vi "sortTimes.vi"(8 "error in (no error)":errorcluster, 10 "Array":T2(array[cluster]), 11 "ScriptEventList in":refnum<class "ScriptEventList.lvclass">) -> (0 "error out":errorcluster, 2 "sortedData":T1, 3 "ScriptEventList out":refnum<class "ScriptEventList.lvclass">)   [LabVIEW 2009, in "Tools.lvlib" / "Scripting.lvlib" / "ScriptEventList.lvclass"]
uses:
  ScriptEventList.lvclass
  DatabaseHelpers/Database Objects/Channel/Channel.lvclass
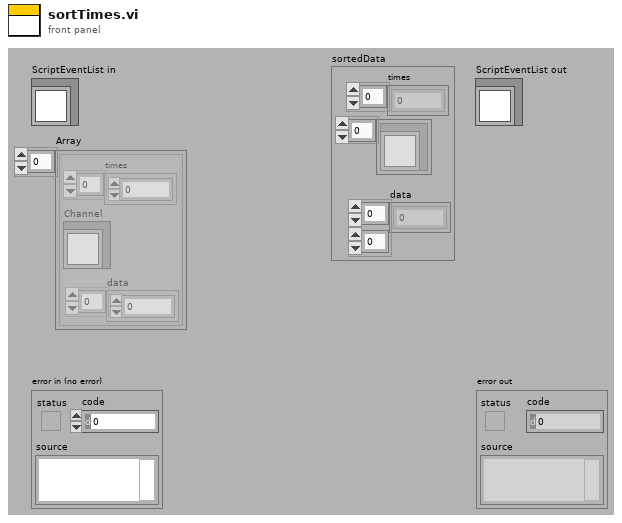
[diagram p1: front panel]
types:
  T1 = cluster{"times":dbl[], refnum<class "Channel.lvclass">[], "data":dbl[][]}
  T2 = cluster{"times":dbl[], "Channel":refnum<class "Channel.lvclass">, "data":dbl[]}[]
  T3 = cluster{dbl[], refnum<class "Channel.lvclass">[], dbl[][]}
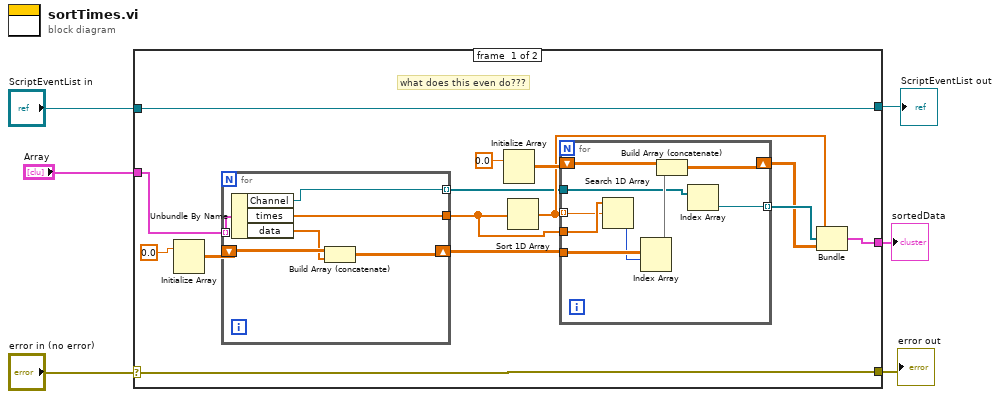
[diagram p0: block diagram]
diagram:
  n1 = case shown="No Error" "error in (no error)" {
    selector: "error in (no error)" -> [w19 w37]
    tunnel: [w19 w37] -> w5
    tunnel: [w20 w36] -> w3
    tunnel: "ScriptEventList in" -> [w20 w36]
    tunnel: "Array" -> [w10 _]
    tunnel: [w11 _] -> w1
    frame #0 {
      # "what does this even do???"
      n2 = Initialize Array(0.0) -> (w18:dbl[][])  [unwired: 2 in]
      n3 = for {
        tunnel: w10 -> [w35] mode=indexing
        shift-right: [w34] -> w16
        shift-left: w18 -> [w33]
        tunnel: [w31] -> w9
        tunnel: [w30] -> w7 mode=indexing
        n4 = Unbundle By Name(w35) -> ("Channel"=w30:refnum<class "Channel.lvclass">, "times"=w31:dbl[], "data"=w32:dbl[])
        n5 = Build Array (concatenate)(w33, w32) -> (w34:dbl[][])
      }
      n6 = Initialize Array(0.0) -> (w15:dbl[][])  [unwired: 2 in]
      n7 = Sort 1D Array(array=w9) -> (sorted array=w8:dbl[])
      n8 = for {
        shift-right: [w27] -> w12
        shift-left: w15 -> [w26]
        tunnel: w16 -> [w29]
        tunnel: w7 -> [w25]
        tunnel: [w24] -> w13 mode=indexing
        tunnel: w8 -> [w21] mode=indexing
        tunnel: w9 -> [w22]
        n9 = Search 1D Array(1D array=w22, element=w21) -> (index of element=w23:i32)  [unwired: 1 in]
        n10 = Index Array(array=w29, index (row)=w23) -> (element=w28:dbl[])  [unwired: 1 in]
        n11 = Build Array (concatenate)(w26, w28) -> (w27:dbl[][])
        n12 = Index Array(array=w25) -> (element=w24:refnum<class "Channel.lvclass">)  [unwired: 1 in]
      }
      n13 = Bundle(w8, w13, w12) -> (w11:T3)  [unwired: 1 in]
    }
    frame #1 {
    }
  }
  "error out" <- w5
  "ScriptEventList out" <- w3
  "sortedData" <- w1
